vi "TrainerLabVIEW.vi"() -> ()   [LabVIEW 2021]
uses:
  <vilib>/Instr/_visa.llb/VISA Configure Serial Port (Instr).vi
panel:
  in  "Color Box":u32(colorbox)
  in  "Slide":dbl(slide) scale=0.0..10.0
  in  "OK Button":bool
  out "Meter":dbl(knob) scale=0.0..10.0
  out "Status indicator":bool
  out "Boolean 2":bool
  out "Boolean":bool
  out "concatenated string":string
  out "Numeric":i32
  out "return count 3":u32
  out "return count 2":u32
  out "read buffer":string
  out "return count":u32
  out "Motor":string
  out "Sensor":string
  out "Type":string
  out "Name":string
  out "read buffer 3":string
  out "Serial Settings:Number of Bytes at Serial Port 2":u32
  out "read buffer 2":string
  in  "VISA resource name 2":refnum<visa-resource-name>
  out "Value":dbl
  in  "Motor":dbl(slide) scale=0.0..180.0
  in  "Done":bool
  in  "Train":bool
  # "Green button that says connected"
  # "help button pops up a help message"
  # "big button to connect - Green light to indicate connection"
  # "move the LED to the top to show connection"
  # "Connect"
  # "Make it go back to this screen when nothing is connected"
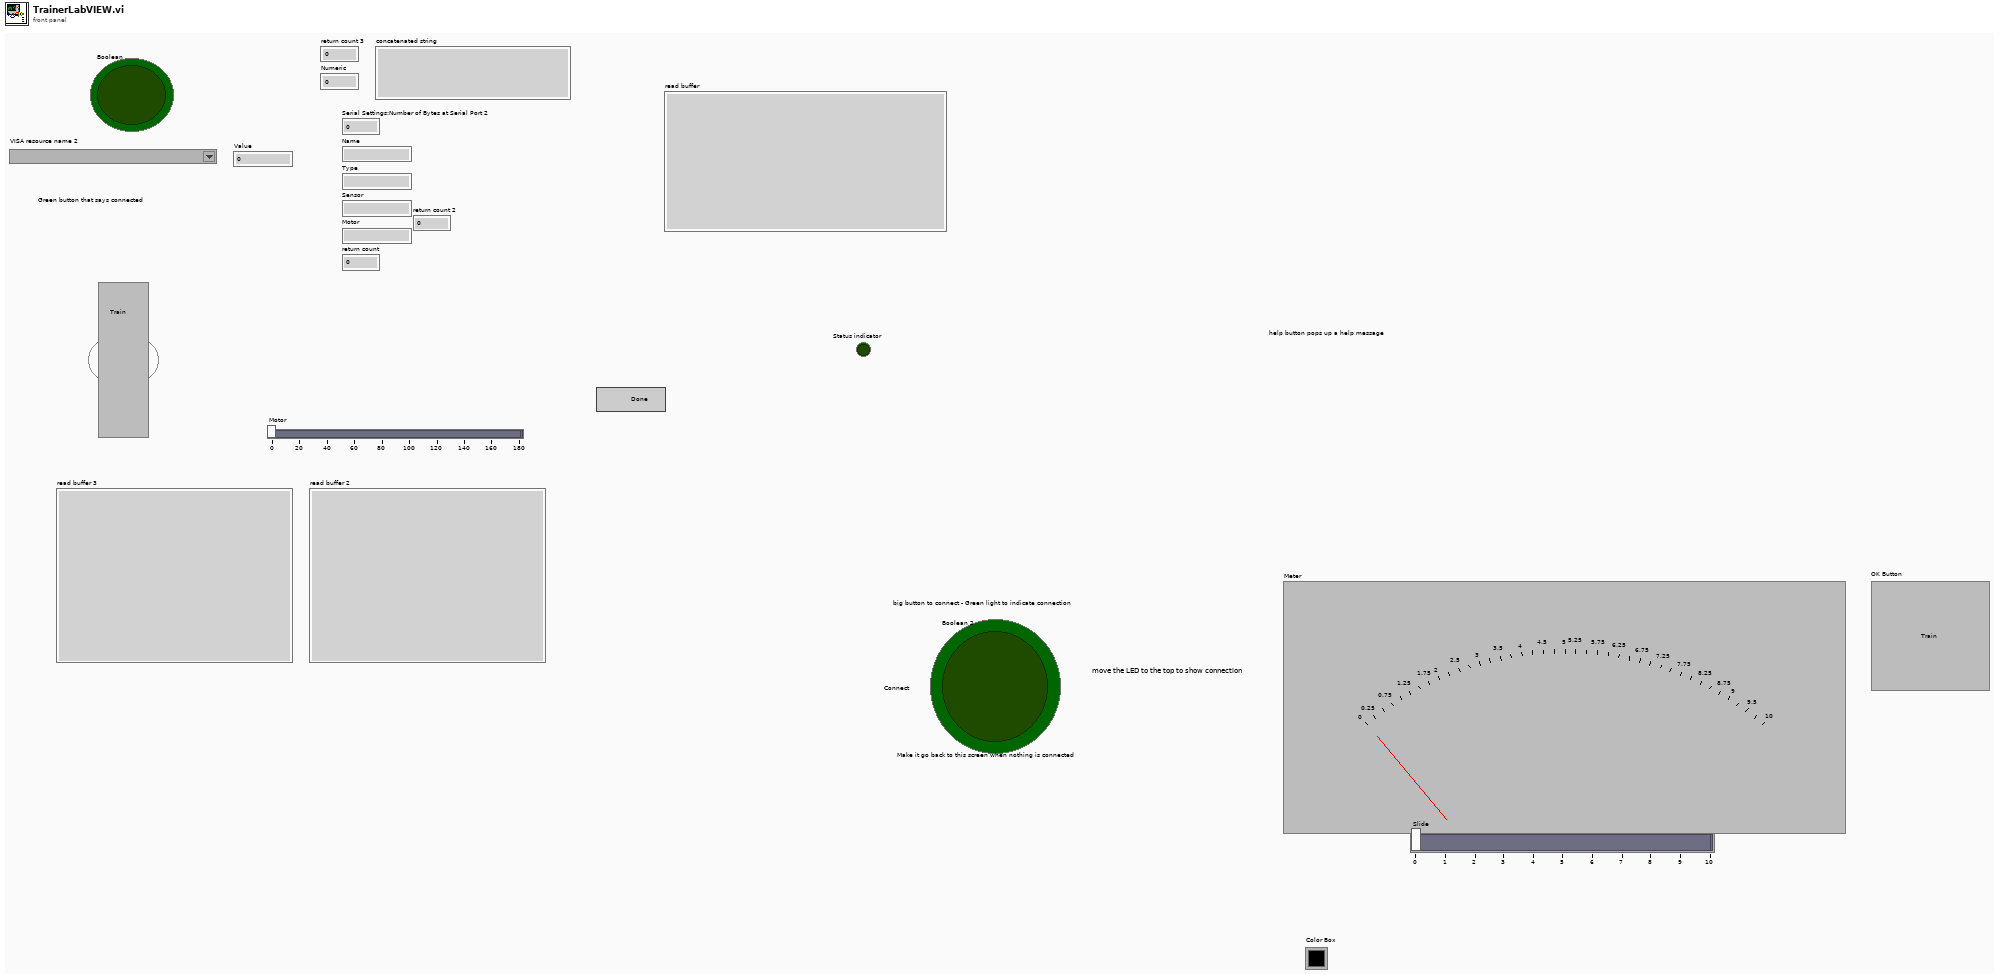
[diagram p1: front panel]
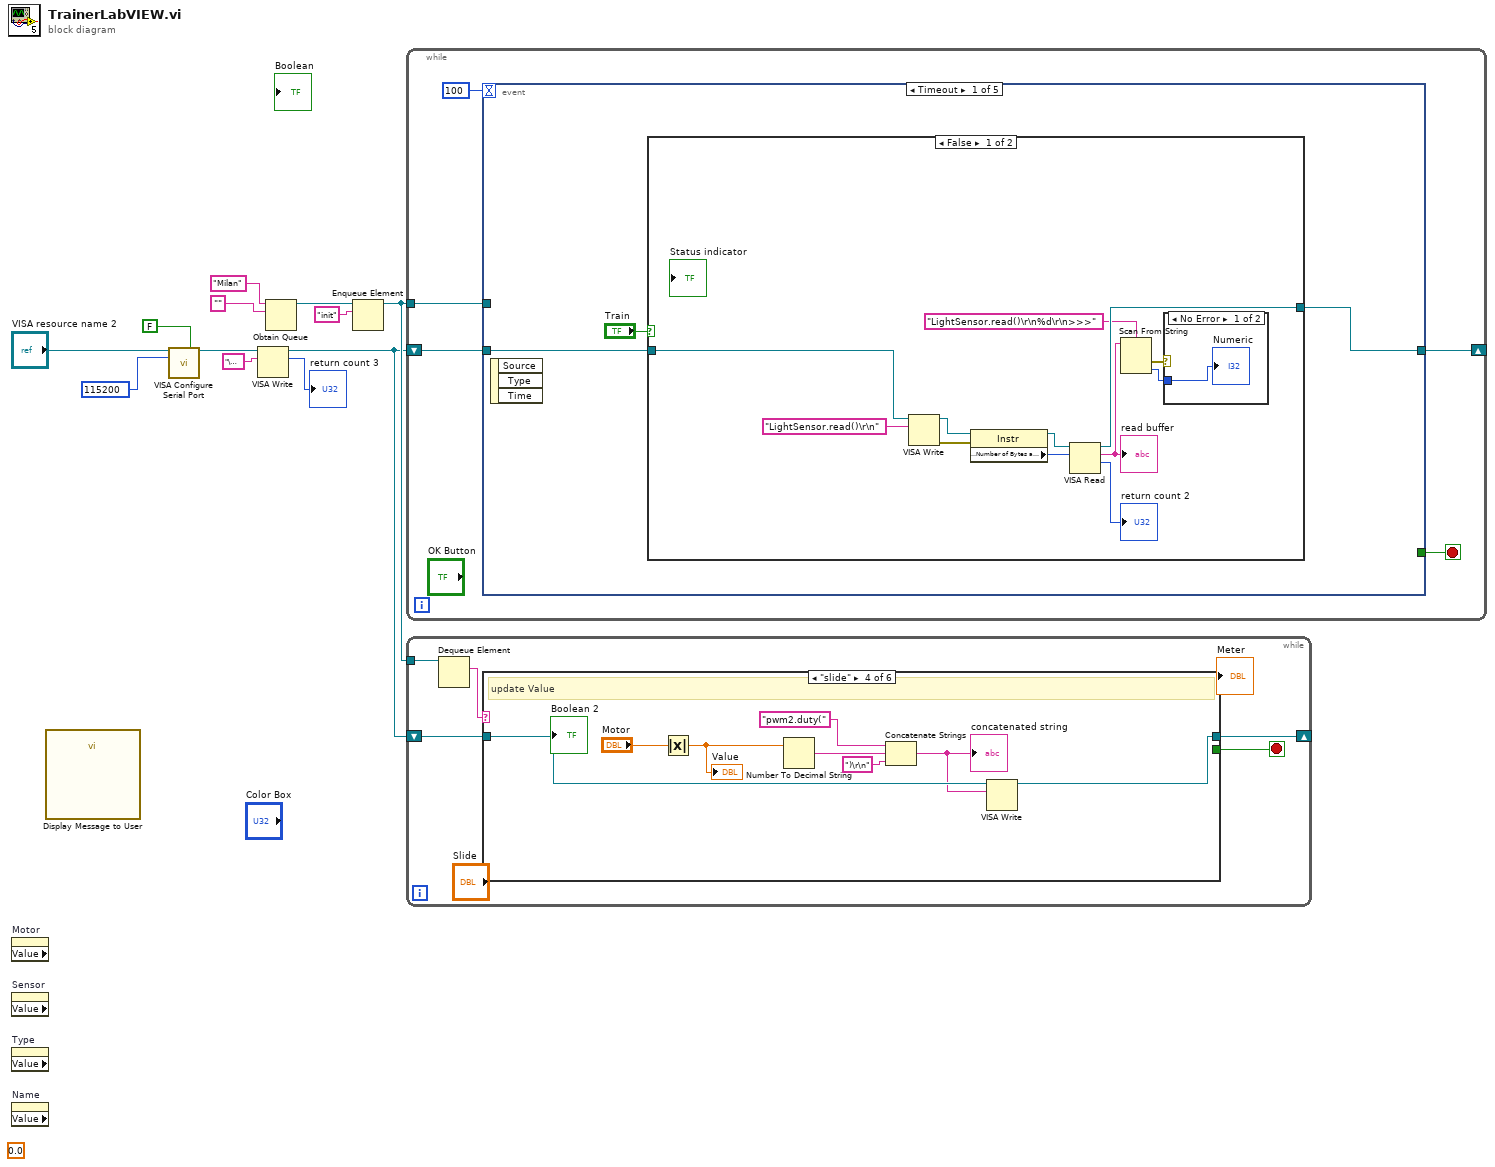
[diagram p0: block diagram]
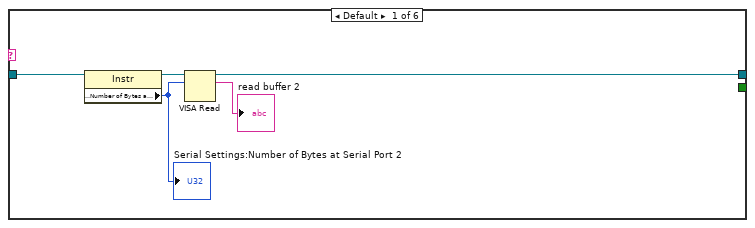
[diagram p2: hidden frame]
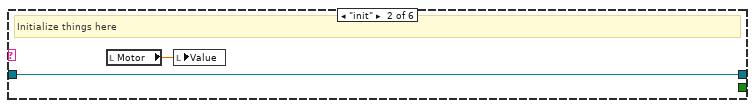
[diagram p3: hidden frame]
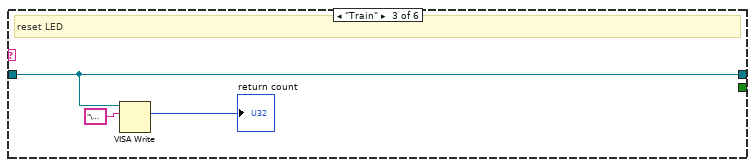
[diagram p4: hidden frame]
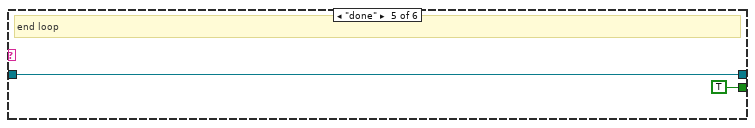
[diagram p5: hidden frame]
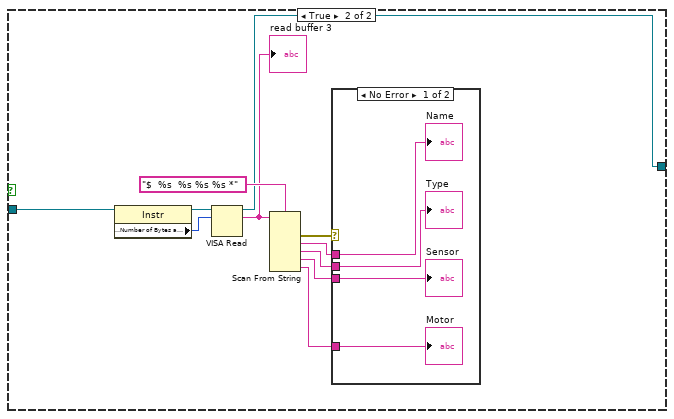
[diagram p8: hidden frame]
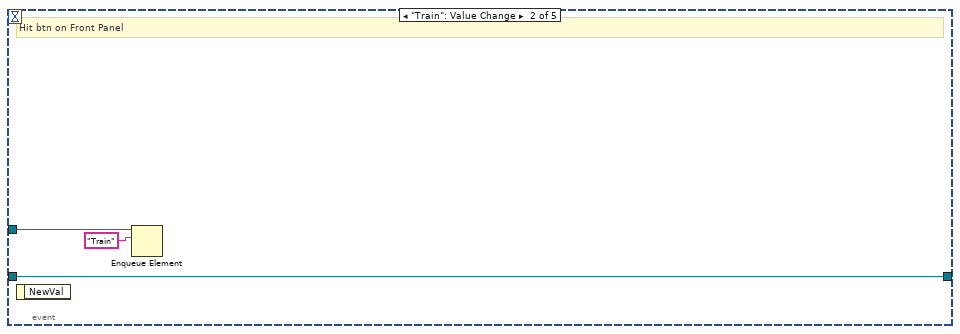
[diagram p10: hidden frame]
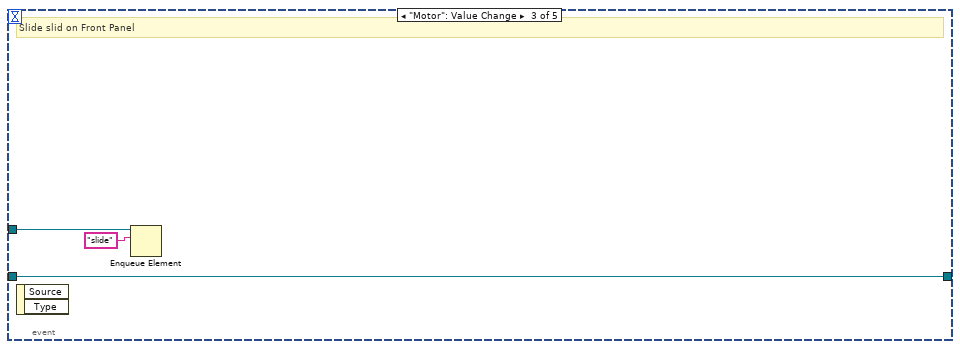
[diagram p11: hidden frame]
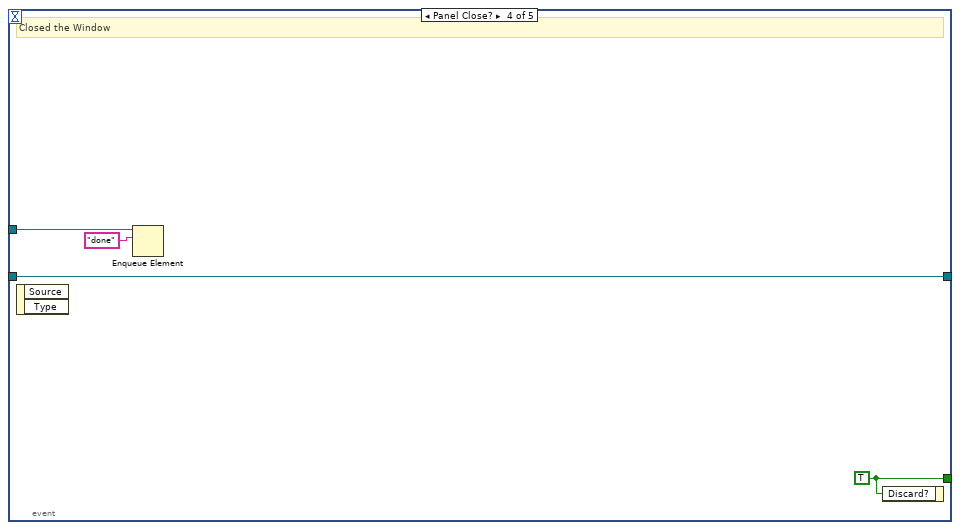
[diagram p12: hidden frame]
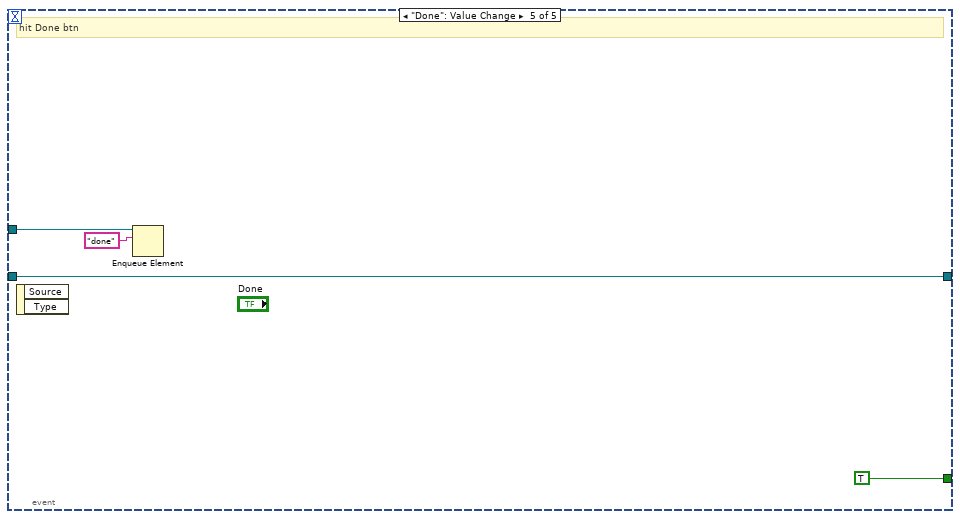
[diagram p13: hidden frame]
diagram:
  (unwired) 0.0
  n1 = property on="Motor" class="Str" props=["Value"]() -> ()  [unwired: 2 in, 3 out]
  n2 = property on="Sensor" class="Str" props=["Value"]() -> ()  [unwired: 2 in, 3 out]
  n3 = property on="Type" class="Str" props=["Value"]() -> ()  [unwired: 2 in, 3 out]
  n4 = property on="Name" class="Str" props=["Value"]() -> ()  [unwired: 2 in, 3 out]
  n5 = call "Display Message to User"() -> ()  [unwired: 10 in, 2 out]
  n6 = call-poly "VISA Configure Serial Port"("VISA resource name"="VISA resource name 2", "Enable Termination\nChar (T)"=FALSE ("Enable Termination\nChar (T)"), "baud rate (9600)"=u32 115200) -> ("VISA resource name out"=w4:refnum<visa-resource-name>)  [unwired: 11 in, 1 out]
  n7 = VISA Write(VISA resource name=w4, write buffer="\u0004") -> (VISA resource name out=w2:refnum<visa-resource-name>, return count=→"return count 3":u32)  [unwired: 1 in, 1 out]
  n8 = Obtain Queue(name (unnamed)="Milan", element data type="") -> (queue out=w12:refnum<queue>)  [unwired: 3 in, 2 out]
  n9 = Enqueue Element(queue=w12, element="init") -> (queue out=w8:refnum<queue>)  [unwired: 2 in, 2 out]
  n10 = while {
    tunnel: w8 -> [w17]
    shift-right: [w14] -> _
    shift-left: w2 -> [w15]
    stop <- w16 stop-if-true
    n11 = event shown="[0] Timeout" {
      selector: _ -> [_ _ _ _ _]
      dyn-events: _ -> [_ _ _ _ _]
      timeout: 100 -> [_ _ _ _ _]
      tunnel: w17 -> [_ w50 w53 w57 w61]
      tunnel: [_ _ _ w56 TRUE ("Discard?")] -> w16
      tunnel: w15 -> [w18 w49 w52 w55 w59]
      tunnel: [w19 w49 w52 w55 w59] -> w14
      event Timeout {
        n12 = event-data() -> ()  [unwired: 1 in, 3 out]
        n13 = case shown="False" "Train" {
          tunnel: w18 -> [w32 w35]
          tunnel: [w27 w37] -> w19
          frame False {
            n14 = VISA Write(VISA resource name=w32, write buffer="LightSensor.read()\r\n") -> (VISA resource name out=w30:refnum<visa-resource-name>, error out=w25:errorcluster)  [unwired: 1 in, 1 out]
            n15 = property class="Instr"(reference=w30, error in=w25) -> (reference out=w29:refnum<visa-resource-name>, "Serial Settings:Number of Bytes at Serial Port"=w28:u32)  [unwired: 1 out]
            n16 = VISA Read(VISA resource name=w29, byte count=w28) -> (VISA resource name out=w27:refnum<visa-resource-name>, read buffer=w21:string, return count=→"return count 2":u32)  [unwired: 1 in, 1 out]
            "read buffer" <- w21
            n17 = Scan From String(format string="LightSensor.read()\r\n%d\r\n>>>", input string=w21) -> (error out=w24:errorcluster, output 1=w23:i32)  [unwired: 3 in, 2 out]
            n18 = case shown="No Error" w24 {
              tunnel: w23 -> [w33 _]
              frame No Error {
                "Numeric" <- w33
              }
              frame Error {
              }
            }
          }
          frame True {
            n19 = property class="Instr"(reference=w35) -> (reference out=w34:refnum<visa-resource-name>, "Serial Settings:Number of Bytes at Serial Port"=w36:u32)  [unwired: 1 in, 1 out]
            n20 = VISA Read(VISA resource name=w34, byte count=w36) -> (VISA resource name out=w37:refnum<visa-resource-name>, read buffer=w38:string)  [unwired: 1 in, 2 out]
            "read buffer 3" <- w38
            n21 = Scan From String(format string="$  %s  %s %s %s *", input string=w38) -> (error out=w44:errorcluster, output 1=w40:string, output 2=w41:string, output 3=w42:string, output 4=w43:string)  [unwired: 6 in, 2 out]
            n22 = case shown="No Error" w44 {
              tunnel: w40 -> [w48 _]
              tunnel: w41 -> [w47 _]
              tunnel: w42 -> [w46 _]
              tunnel: w43 -> [w45 _]
              frame No Error {
                "Name" <- w48
                "Type" <- w47
                "Sensor" <- w46
                "Motor" <- w45
              }
              frame Error {
              }
            }
          }
        }
      }
      event "Train": Value Change {
        # "Hit btn on Front Panel"
        n23 = event-data() -> ()  [unwired: 1 in, 1 out]
        n24 = Enqueue Element(queue=w50, element="Train") -> ()  [unwired: 2 in, 3 out]
      }
      event "Motor": Value Change {
        # "Slide slid on Front Panel"
        n25 = event-data() -> ()  [unwired: 1 in, 2 out]
        n26 = Enqueue Element(queue=w53, element="slide") -> ()  [unwired: 2 in, 3 out]
      }
      event Panel Close? {
        w56 = TRUE ("Discard?")
        # "Closed the Window"
        n27 = event-data() -> ()  [unwired: 1 in, 2 out]
        n28 = Enqueue Element(queue=w57, element="done") -> ()  [unwired: 2 in, 3 out]
        n29 = event-data("Discard?"=w56) -> ()  [unwired: 1 in, 1 out]
      }
      event "Done": Value Change {
        # "hit Done btn"
        n30 = event-data() -> ()  [unwired: 1 in, 2 out]
        n31 = Enqueue Element(queue=w61, element="done") -> ()  [unwired: 2 in, 3 out]
      }
    }
  }
  n32 = while {
    tunnel: w8 -> [w67]
    shift-right: [w63] -> _
    shift-left: w2 -> [w64]
    stop <- w65 stop-if-true
    n33 = Dequeue Element(queue=w67) -> (element=w66:string)  [unwired: 2 in, 3 out]
    n34 = case shown="\"slide\"" w66 {
      tunnel: [_ _ _ _ TRUE ("Discard?") _] -> w65
      tunnel: w64 -> [w69 w73 w77 w85 w86 w88]
      tunnel: [w68 w73 w77 w79 w86 w88] -> w63
      frame Default {
        n35 = property class="Instr"(reference=w69) -> (reference out=w70:refnum<visa-resource-name>, "Serial Settings:Number of Bytes at Serial Port"=w71:u32)  [unwired: 1 in, 1 out]
        "Serial Settings:Number of Bytes at Serial Port 2" <- w71
        n36 = VISA Read(VISA resource name=w70, byte count=w71) -> (VISA resource name out=w68:refnum<visa-resource-name>, read buffer=→"read buffer 2":string)  [unwired: 1 in, 2 out]
      }
      frame "init" {
        # "Initialize things here"
        n37 = local read "Motor"() -> (w74:dbl)
        n38 = local write "Value"(w74) -> ()
      }
      frame "Train" {
        # "reset LED"
        n39 = VISA Write(VISA resource name=w77, write buffer="\u0003") -> (return count=→"return count":u32)  [unwired: 1 in, 2 out]
      }
      frame "slide" {
        # "update Value"
        n40 = Absolute Value(x="Motor") -> (abs(x)=w78:dbl)
        "Value" <- w78
        n41 = Number To Decimal String(number=w78) -> (decimal integer string=w82:string)  [unwired: 1 in]
        n42 = Concatenate Strings("pwm2.duty(", w82, ")\r\n" ("string")) -> (w80:string)
        "concatenated string" <- w80
        n43 = VISA Write(VISA resource name=w85, write buffer=w80) -> (VISA resource name out=w79:refnum<visa-resource-name>)  [unwired: 1 in, 2 out]
      }
      frame "done" {
        # "end loop"
      }
      frame "" {
      }
    }
  }
